vi "Excel Write Table.vi"(4 "행헤더":string[](array[string]), 5 "Address":cluster{"Row":i32, "Column":i32}={"Row"=1, "Column"=1}, 6 "열헤더":string[](array[string]), 7 "show grid lines":bool=TRUE, 8 "error in":errorcluster caption="에러 입력(에러 없음)", 10 "table":string[][](table), 11 "report in":refnum<class "NI_report.lvclass">) -> (0 "error out":errorcluster caption="에러 출력", 1 "Range out":refnum<k7>, 2 "worksheet out":refnum<k7>, 3 "report out":refnum<class "NI_report.lvclass">)   [LabVIEW 2020]
uses:
  <vilib>/Utility/NIReport.llb/NI_report.lvclass
  <vilib>/addons/_office/NI_ReportGenerationToolkit.lvlib
  <vilib>/Utility/NIReport.llb/Excel/NI_Excel.lvclass
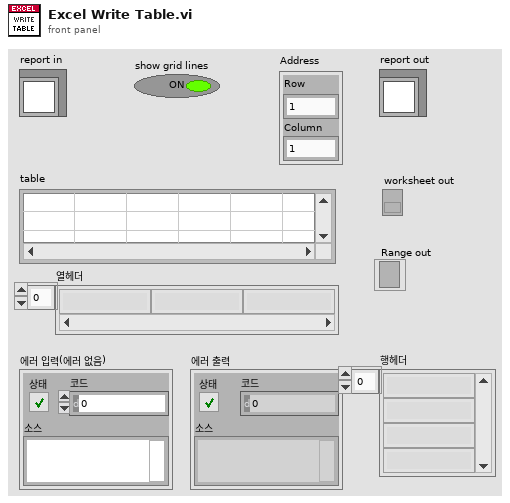
[diagram p1: front panel]
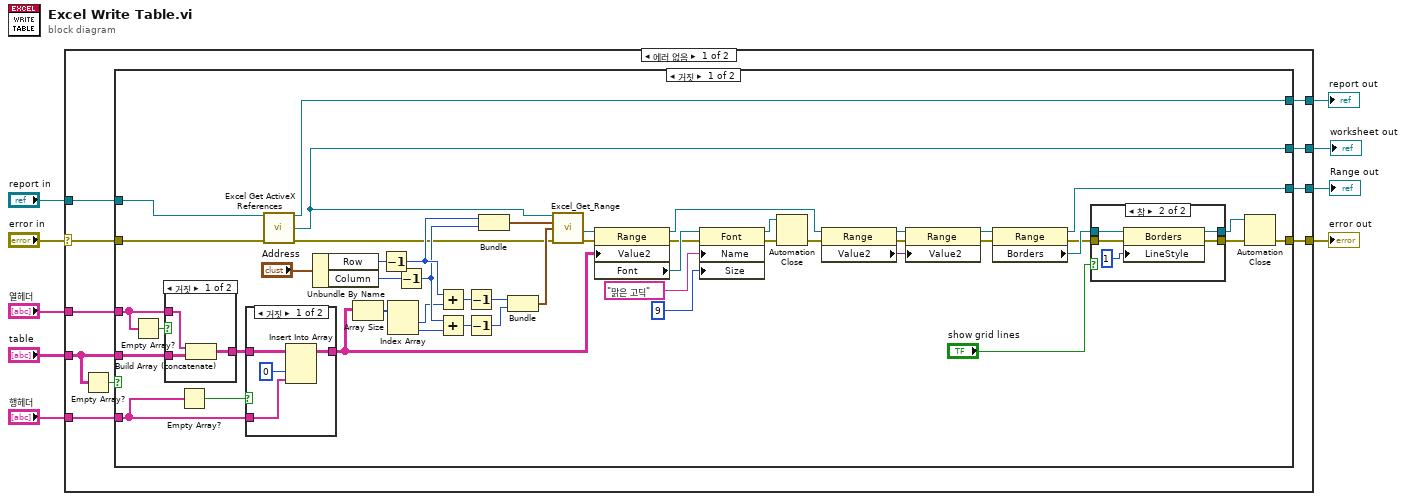
[diagram p0: block diagram]
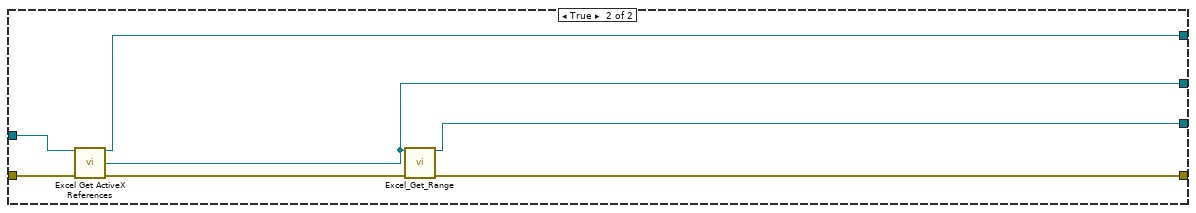
[diagram p5: hidden frame]
diagram:
  n1 = case shown="에러 없음" "error in" {
    selector: "error in" -> [w13 w92]
    tunnel: [w19 w92] -> w9
    tunnel: [w18 w91] -> w8
    tunnel: "report in" -> [w17 w91]
    tunnel: [w16 _] -> w6
    tunnel: [w15 _] -> w5
    tunnel: "열헤더" -> [w14 _]
    tunnel: "table" -> [w12 _]
    tunnel: "행헤더" -> [w10 _]
    frame No Error {
      n2 = Empty Array?(array=w12) -> (empty?=w11:bool)
      n3 = case shown="거짓" w11 {
        tunnel: w12 -> [w67 _]
        tunnel: w13 -> [w66 w90]
        tunnel: [w65 w86] -> w19
        tunnel: [w64 w89] -> w18
        tunnel: w17 -> [w63 w88]
        tunnel: [w62 w87] -> w16
        tunnel: [w61 w85] -> w15
        tunnel: w14 -> [w60 _]
        tunnel: w10 -> [w22 _]
        frame False {
          n4 = Empty Array?(array=w60) -> (empty?=w35:bool)
          n5 = case shown="거짓" w35 {
            tunnel: w67 -> [w75 w76]
            tunnel: [w74 w76] -> w23
            tunnel: w60 -> [w73 _]
            frame False {
              n6 = Build Array (concatenate)(w73, w75) -> (w74:string[][])
            }
            frame True {
            }
          }
          n7 = Empty Array?(array=w22) -> (empty?=w20:bool)
          n8 = case shown="거짓" w20 {
            tunnel: w23 -> [w71 w72]
            tunnel: w22 -> [w69 _]
            tunnel: [w68 w72] -> w21
            frame False {
              n9 = Insert Into Array(array=w71, index (col)=0 ("비활성화된 인덱스 (열)"), new element=w69) -> (w68:string[][])  [unwired: 1 in]
            }
            frame True {
            }
          }
          n10 = call <vilib>:"Excel Get ActiveX References.vi"("report in"=w63, "error in (no error)"=w66) -> ("report out"=w64:refnum<class "NI_report.lvclass">, "Excel._Worksheet"=w62:refnum<k7>, "error out"=w36:errorcluster)  [unwired: 7 in, 4 out]
          n11 = Unbundle By Name("Address") -> ("Row"=w40:i32, "Column"=w39:i32)
          n12 = Array Size(array=w21) -> (size(s)=w59:i32[])
          n13 = Decrement(x=w40) -> (x-1=w38:i32)
          n14 = Index Array(array=w59) -> (element #1=w24:i32, element #2=w55:i32)  [unwired: 2 in]
          n15 = Decrement(x=w39) -> (x-1=w37:i32)
          n16 = Add(x=w38, y=w24) -> (x+y=w48:i32)
          n17 = Add(x=w37, y=w55) -> (x+y=w47:i32)
          n18 = Decrement(x=w48) -> (x-1=w45:i32)
          n19 = Decrement(x=w47) -> (x-1=w44:i32)
          n20 = Bundle(w38, w37) -> (w49:cluster{i32, i32})  [unwired: 1 out]
          n21 = Bundle(w45, w44) -> (w46:cluster{i32, i32})  [unwired: 1 out]
          n22 = call <vilib>:"Excel_Get_Range.vi"("Excel._Worksheet"=w62, "start"=w49, "end"=w46, "error in (no error)"=w36) -> ("Range"=w58:refnum<k7>, "error out"=w57:errorcluster)  [unwired: 2 in, 8 out]
          n23 = property class="Range"(reference=w58, error in=w57, "Value2"=w21) -> (reference out=w50:refnum<k7>, error out=w28:errorcluster, "Font"=w31:refnum<k7>)
          n24 = property class="Font"(reference=w31, error in=w28, "Name"="맑은 고딕", "Size"=9) -> (reference out=w26:refnum<k7>, error out=w27:errorcluster)
          n25 = Automation Close(3:w27, 5:w26) -> (0:w25:errorcluster)
          n26 = property class="Range"(reference=w50, error in=w25) -> (reference out=w34:refnum<k7>, error out=w33:errorcluster, "Value2"=w32:variant)
          n27 = property class="Range"(reference=w34, error in=w33, "Value2"=w32) -> (reference out=w42:refnum<k7>, error out=w43:errorcluster)
          n28 = property class="Range"(reference=w42, error in=w43) -> (reference out=w61:refnum<k7>, error out=w53:errorcluster, "Borders"=w54:refnum<k7>)
          n29 = case shown="참" "show grid lines" {
            tunnel: w54 -> [w77 w82]
            tunnel: w53 -> [w78 w81]
            tunnel: [w78 w80] -> w52
            tunnel: [w77 w79] -> w51
            frame False {
            }
            frame True {
              n30 = property class="Borders"(reference=w82, error in=w81, "LineStyle"=1) -> (reference out=w79:refnum<k7>, error out=w80:errorcluster)
            }
          }
          n31 = Automation Close(3:w52, 5:w51) -> (0:w65:errorcluster)
        }
        frame True {
          n32 = call <vilib>:"Excel Get ActiveX References.vi"("report in"=w88, "error in (no error)"=w90) -> ("report out"=w89:refnum<class "NI_report.lvclass">, "Excel._Worksheet"=w87:refnum<k7>, "error out"=w84:errorcluster)  [unwired: 7 in, 4 out]
          n33 = call <vilib>:"Excel_Get_Range.vi"("Excel._Worksheet"=w87, "error in (no error)"=w84) -> ("Range"=w85:refnum<k7>, "error out"=w86:errorcluster)  [unwired: 4 in, 8 out]
        }
      }
    }
    frame Error {
    }
  }
  "error out" <- w9
  "report out" <- w8
  "worksheet out" <- w6
  "Range out" <- w5
